vi "TEST_Main_decode.vi"() -> ()   [LabVIEW 2021]
panel:
  out "mesage_bits":string
  out "secret_ message":string
  in  "Bits_modified":string(combo)
  out "Original":T1(plugin-control)
  # "Secret decode VI"
  # "Overview: This VI separates RGB planes from a given color image tand reads the defined LSB of the RED PLANE  to decode the hidden message within the input image.\n\nInstructions:\n1. Make sure you update the path of the image.\n2. Select the number of encoded bits\n3. Run the VI\n4.Check the message.\n\n\nAuthor: Jaime Burbano V\nLast Modified: 2022-06-10"
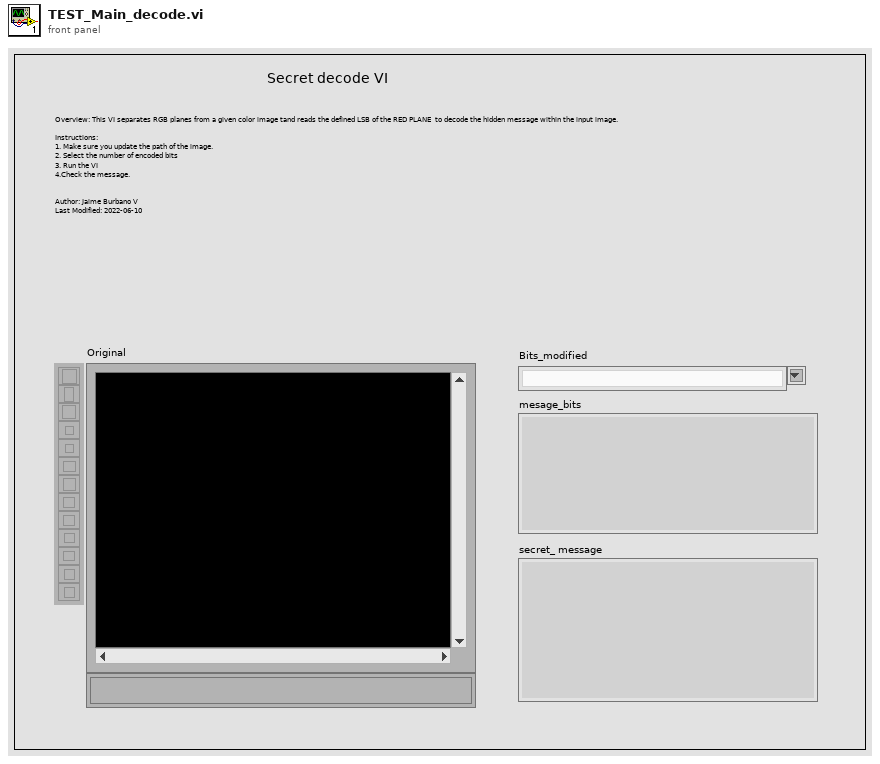
[diagram p1: front panel]
types:
  T1 = typedef "IMAQ Image.ctl" = refnum<image>
  T2 = typedef "Image Type" = u32
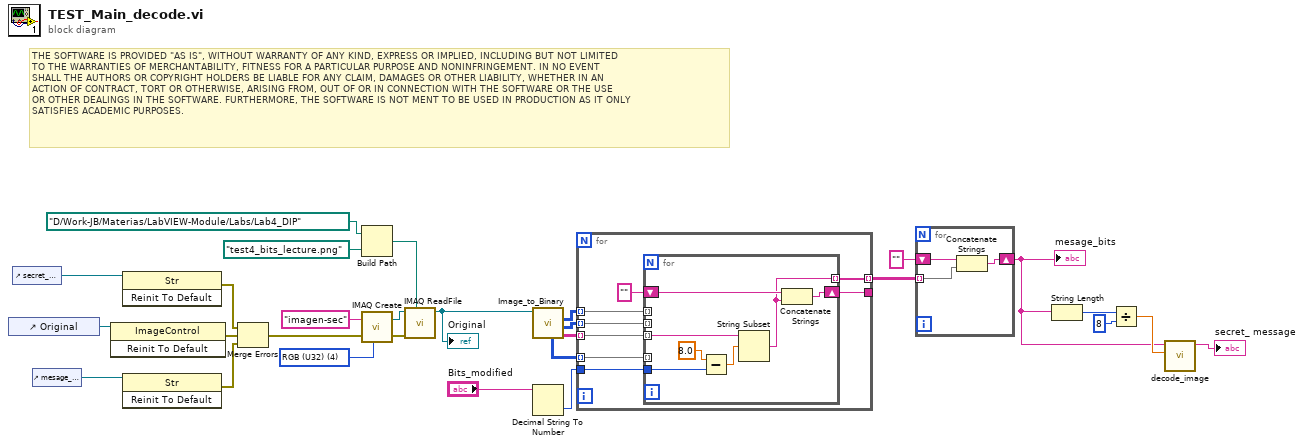
[diagram p0: block diagram]
diagram:
  w26 = T2 4 items=["Grayscale (U8)", "Grayscale (I16)", "Grayscale (SGL)", "Complex (CSG)", "RGB (U32)", "HSL (U32)", "RGB (U64)", "Grayscale (U16)"] ("Image Type")
  # "THE SOFTWARE IS PROVIDED \"AS IS\", WITHOUT WARRANTY OF ANY KIND, EXPRESS OR IMPLIED, INCLUDING BUT NOT LIMITED \nTO THE WARRANTIES OF MERCHANTABILITY, FITNESS FOR A PARTICULAR PURPOSE AND NONINFRINGEMENT. IN NO EVENT \nSHALL THE AUTHORS OR COPYRIGHT HOLDERS BE LIABLE FOR ANY CLAIM, DAMAGES OR OTHER LIABILITY, WHETHER IN AN \nACTION OF CONTRACT, TORT OR OTHERWISE, ARISING FROM, OUT OF OR IN CONNECTION WITH THE SOFTWARE OR THE USE \nOR OTHER DEALINGS IN THE SOFTWARE. FURTHERMORE, THE SOFTWARE IS NOT MENT TO BE USED IN PRODUCTION AS IT ONLY \nSATISFIES ACADEMIC PURPOSES."
  n1 = control-ref of="Original"() -> (w9:refnum<vi>)
  n2 = control-ref of="secret_ message"() -> (w10:refnum<vi>)
  n3 = control-ref of="mesage_bits"() -> (w1:refnum<vi>)
  n4 = invoke class="ImageControl" method="Reinit To Default"(reference=w9) -> (error out=w7:errorcluster)  [unwired: 2 in, 2 out]
  n5 = invoke class="Str" method="Reinit To Default"(reference=w10) -> (error out=w8:errorcluster)  [unwired: 2 in, 2 out]
  n6 = invoke class="Str" method="Reinit To Default"(reference=w1) -> (error out=w6:errorcluster)  [unwired: 2 in, 2 out]
  n7 = Merge Errors(w8, w7, w6) -> (w5:errorcluster)
  n8 = Build Path(base path=path "D:/Work-JB/Materias/LabVIEW-Module/Labs/Lab4_DIP", name or relative path=path "test4_bits_lecture.png") -> (appended path=w23:path)
  n9 = call "IMAQ Create"("Image Name"="imagen-sec", "Image Type"=w26, "error in (no error)"=w5) -> ("New Image"=w24:T1, "error out"=w25:errorcluster)  [unwired: 2 in]
  n10 = call "IMAQ ReadFile"("File Path"=w23, "error in (no error)"=w25, "Image"=w24) -> ("Image Out"=w21:T1)  [unwired: 4 in, 4 out]
  "Original" <- w21
  n11 = call "Image_to_Binary.vi"("Image-in"=w21) -> ("Red Binary"=w20:string[][], "Red Number"=w19:u8[][], "Blue Number"=w17:u8[][], "Green Number"=w18:u8[][])  [unwired: 3 in, 4 out]
  n12 = Decimal String To Number(string="Bits_modified") -> (number=w15:i32)  [unwired: 2 in, 1 out]
  n13 = for {
    tunnel: w20 -> [w36] mode=indexing
    tunnel: w19 -> [w35] mode=indexing
    tunnel: w18 -> [w34] mode=indexing
    tunnel: w17 -> [w33] mode=indexing
    tunnel: w15 -> [w32]
    tunnel: [w31] -> _
    tunnel: [w29] -> w4 mode=indexing
    n14 = for {
      tunnel: w36 -> [w40] mode=indexing
      tunnel: w35 -> [_] mode=indexing
      tunnel: w34 -> [_] mode=indexing
      tunnel: w33 -> [_] mode=indexing
      tunnel: w32 -> [w42]
      shift-right: [w38] -> w31
      shift-left: "" -> [w39]
      tunnel: [w37] -> w29 mode=indexing
      n15 = Subtract(x=8.0, y=w42) -> (x-y=w41:dbl)
      n16 = String Subset(string=w40, offset (0)=w41) -> (substring=w37:string)  [unwired: 1 in]
      n17 = Concatenate Strings(w39, w37) -> (w38:string)
    }
  }
  n18 = for {
    tunnel: w4 -> [w44] mode=indexing
    shift-right: [w46] -> w3
    shift-left: "" -> [w45]
    n19 = Concatenate Strings(w45, w44) -> (w46:string)
  }
  "mesage_bits" <- w3
  n20 = String Length(string=w3) -> (length=w14:i32)
  n21 = Divide(x=w14, y=8) -> (x/y=w12:dbl)
  n22 = call "decode_image.vi"("Numeric"=w12, "String in"=w3) -> ("String out"=→"secret_ message":string)  [unwired: 9 in]
